vi "Scripting_GetVIClassDependency.vi"(0 "ViRef":refnum<vi>, 5 "error in (no error)":errorcluster) -> (15 "DepVIs":T1[](array[typedef]), 19 "error out":errorcluster)   [LabVIEW 2016]
uses:
  <resource>/Framework/Providers/Open_GDS/ClassProviders/Common/ScriptingFunctions/Scripting_VIClassDependency.ctl
  <resource>/Framework/Providers/Open_GDS/ClassProviders/Common/ScriptingFunctions/SubVIs/Scripting_ViDependencyType.ctl
  <vilib>/Utility/traverseref.llb/TRef TravTarget.ctl
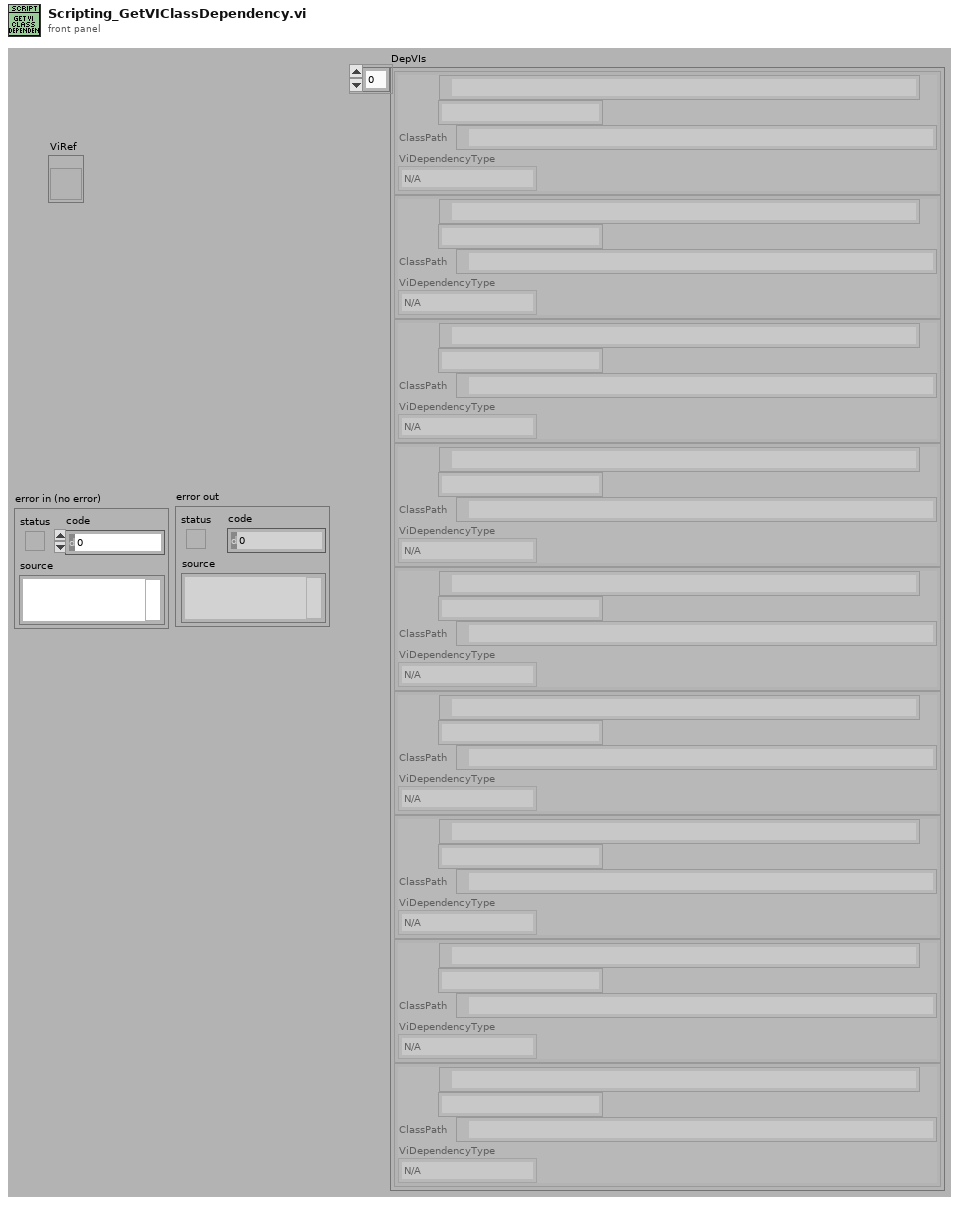
[diagram p1: front panel]
types:
  T1 = typedef "Scripting_VIClassDependency.ctl" = cluster{"VIPath":path, "Class":string, "ClassPath":path, "ViDependencyType":T2}
  T2 = typedef "Scripting_ViDependencyType.ctl" = enum16{"N/A", "Launches"}
  T3 = enum32{"invalid VI type", "Standard VI", "Control VI", "Global VI", "Polymorphic VI", "Configuration VI", "SubSystem", "Facade VI", "Method VI", "Statechart Diagram VI"}
  T4 = enum32{"invalid lock state", "Not Locked", "Locked (No Password)", "Password-protected"}
  T5 = cluster{"ClassControls":refnum<vi>[], "NewClassControl":path, "Diagrams":refnum<vi>[], "DepVIs":T1[]}
  T6 = typedef "TRef TravTarget.ctl" = enum16{"FP", "BD", "Other"}
  T7 = enum32{"not a typedef", "typedef", "strict typedef", "class private data"}
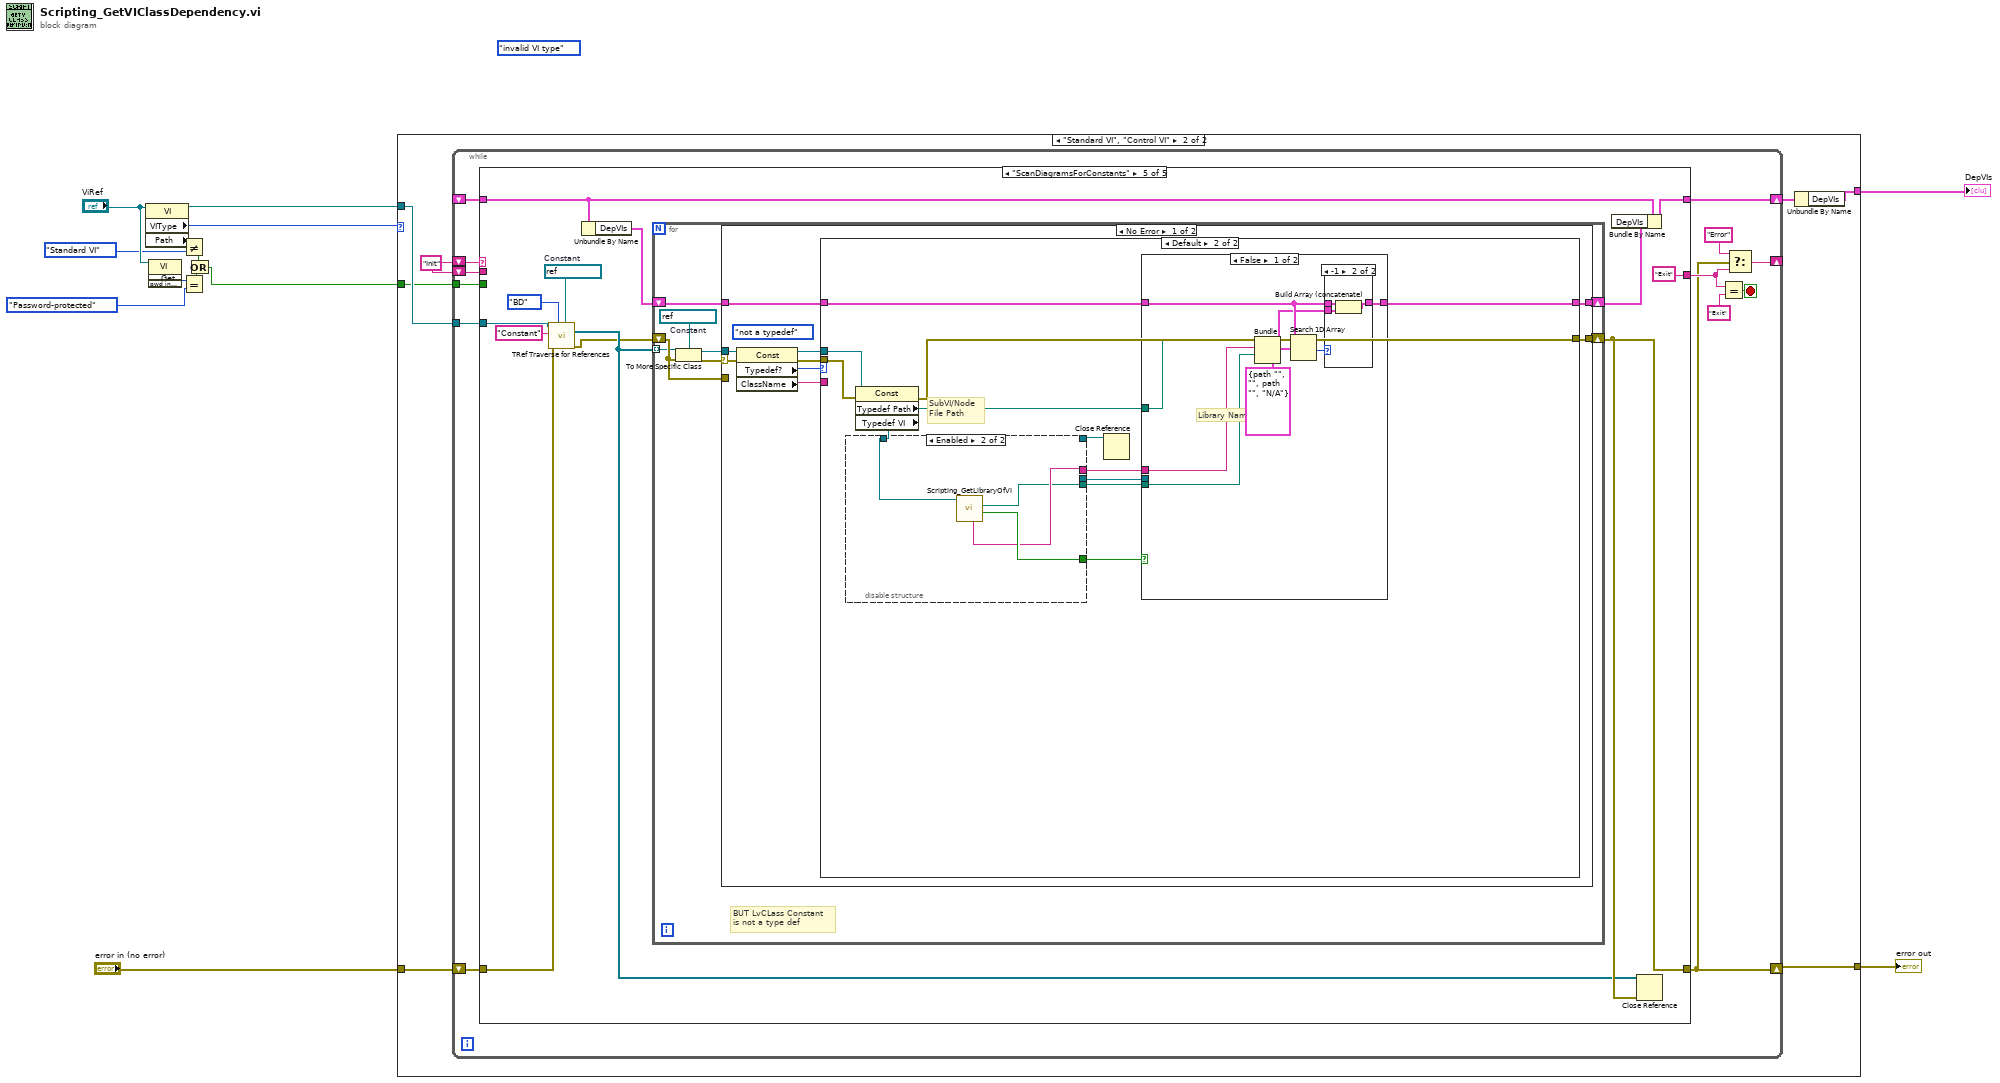
[diagram p0: block diagram]
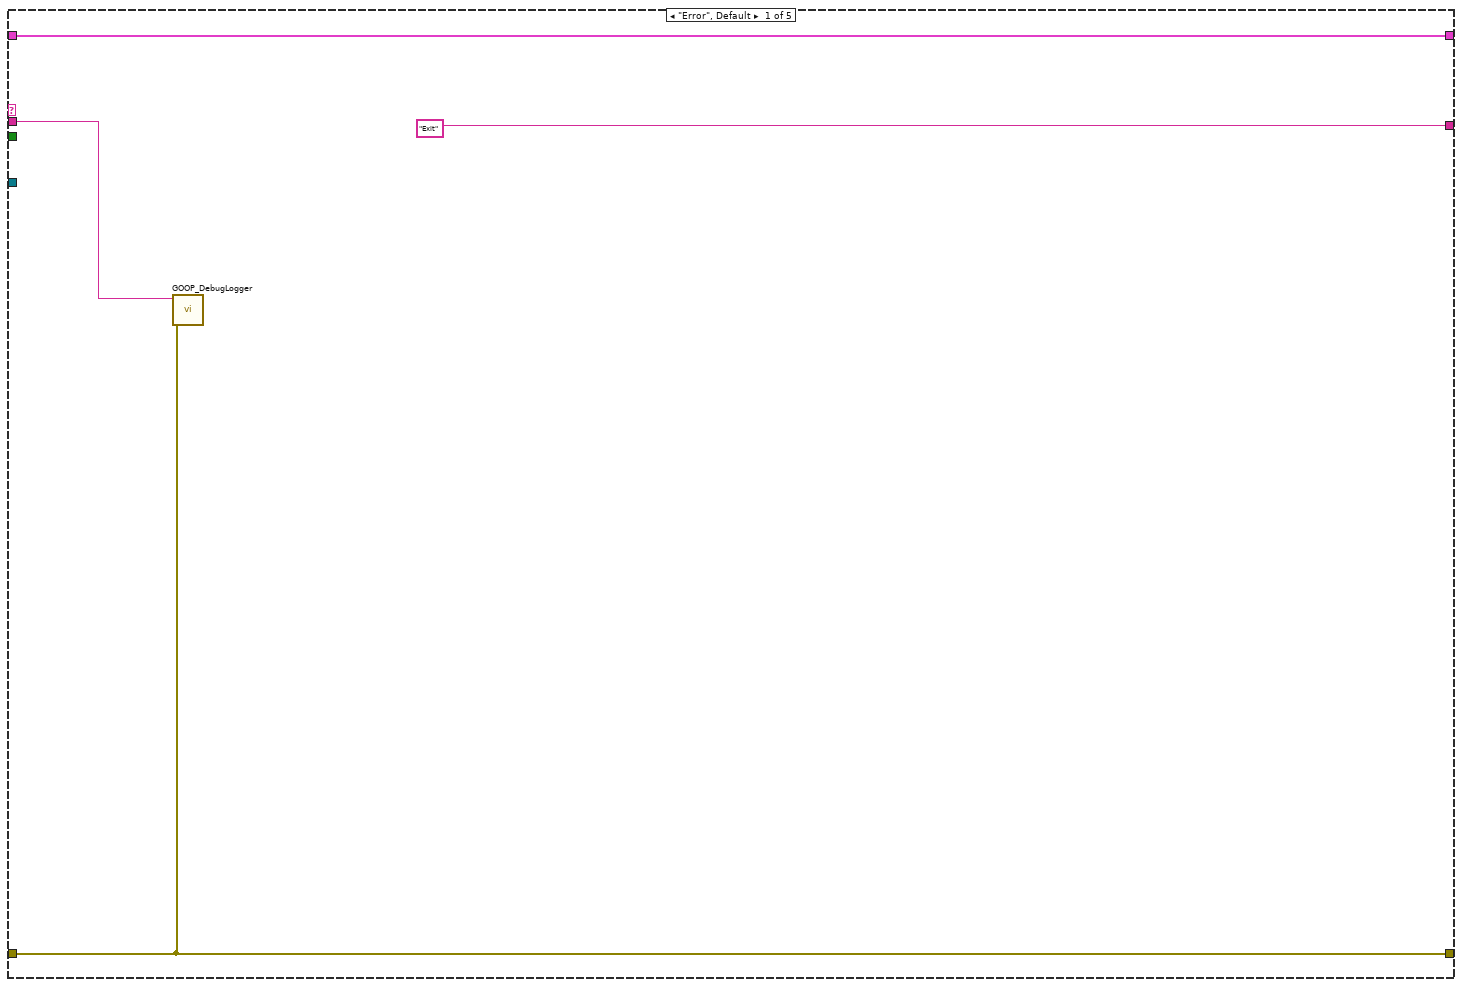
[diagram p3: hidden frame]
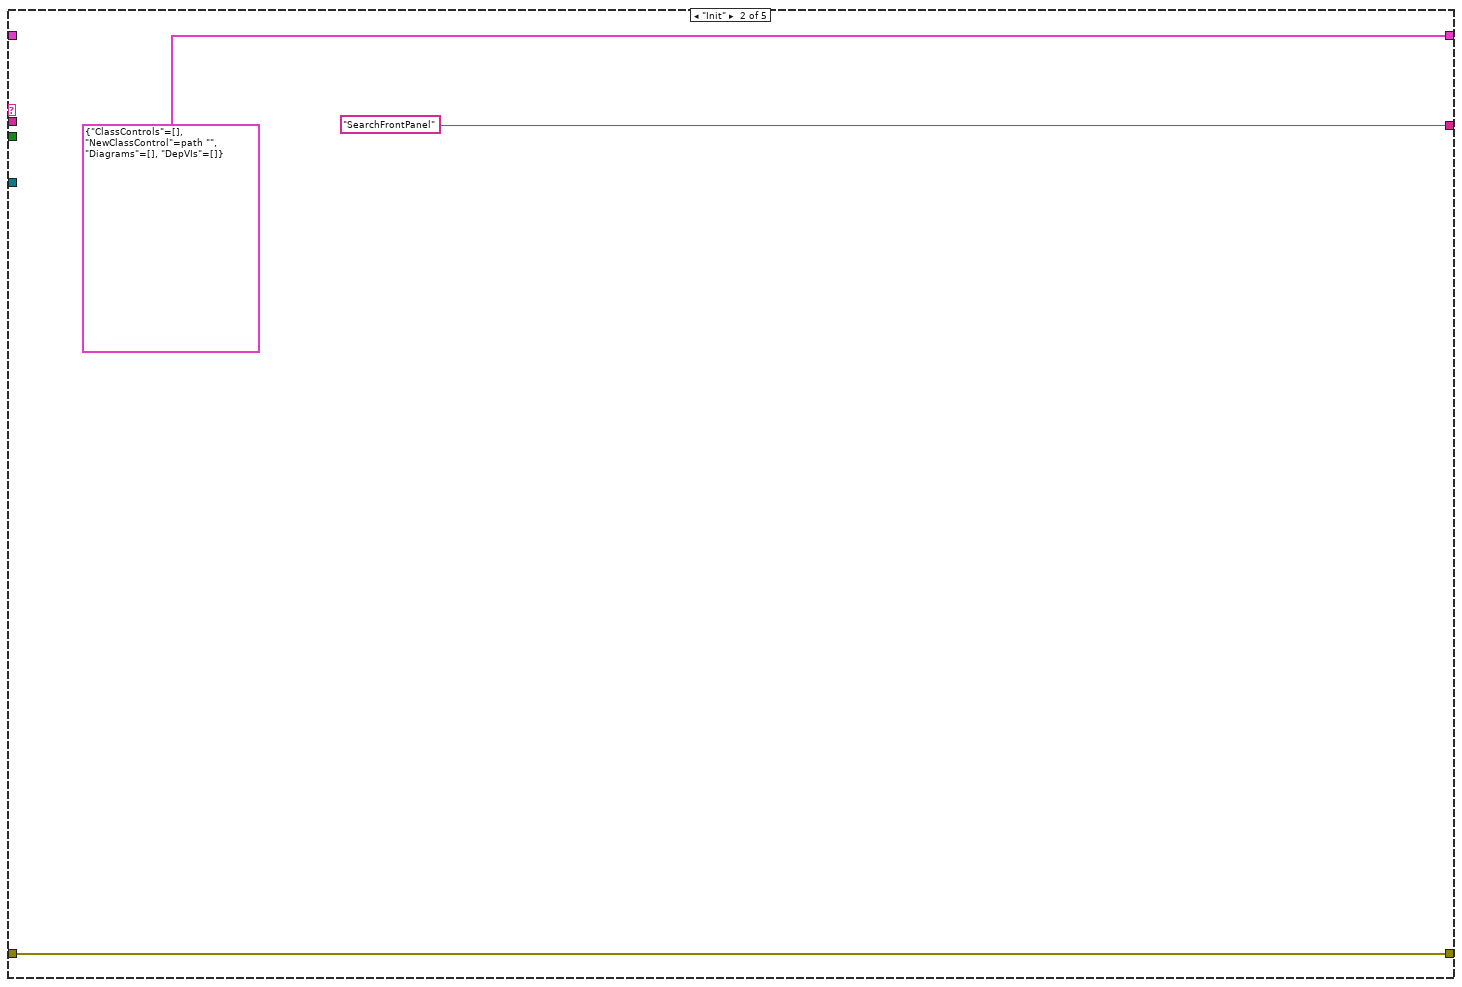
[diagram p4: hidden frame]
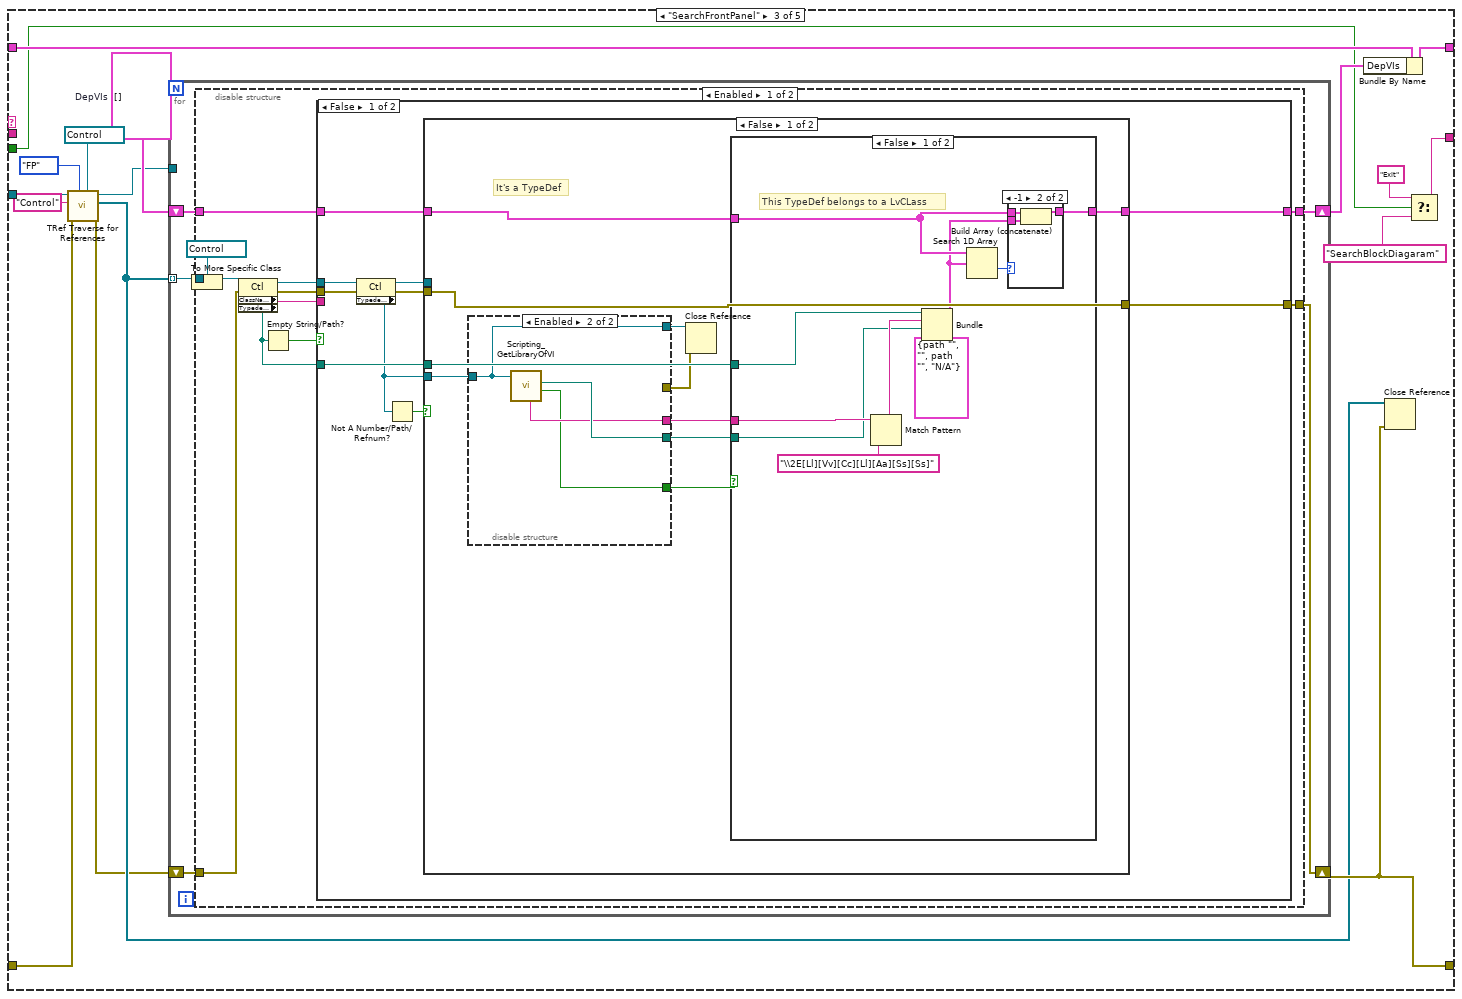
[diagram p5: hidden frame]
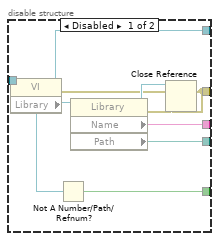
[diagram p6: hidden frame]
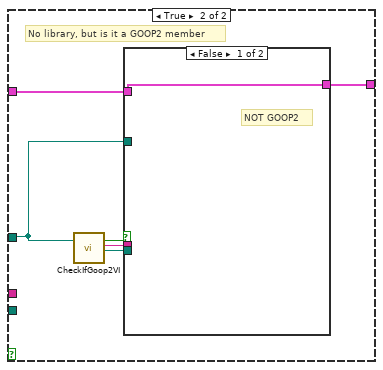
[diagram p8: hidden frame]
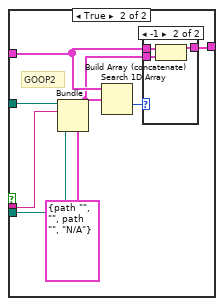
[diagram p9: hidden frame]
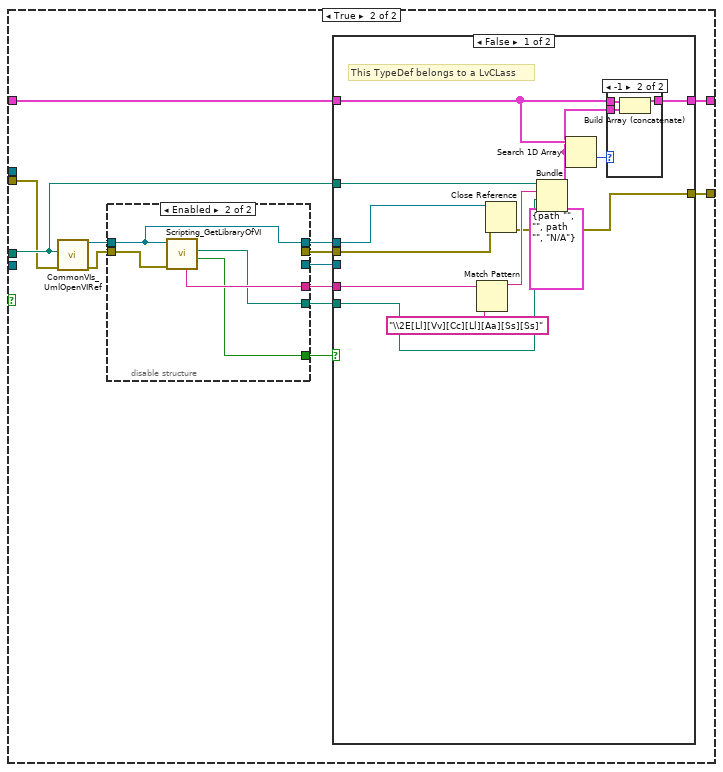
[diagram p11: hidden frame]
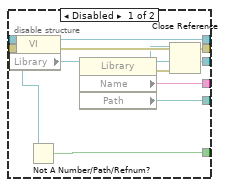
[diagram p12: hidden frame]
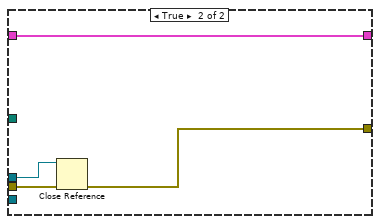
[diagram p14: hidden frame]
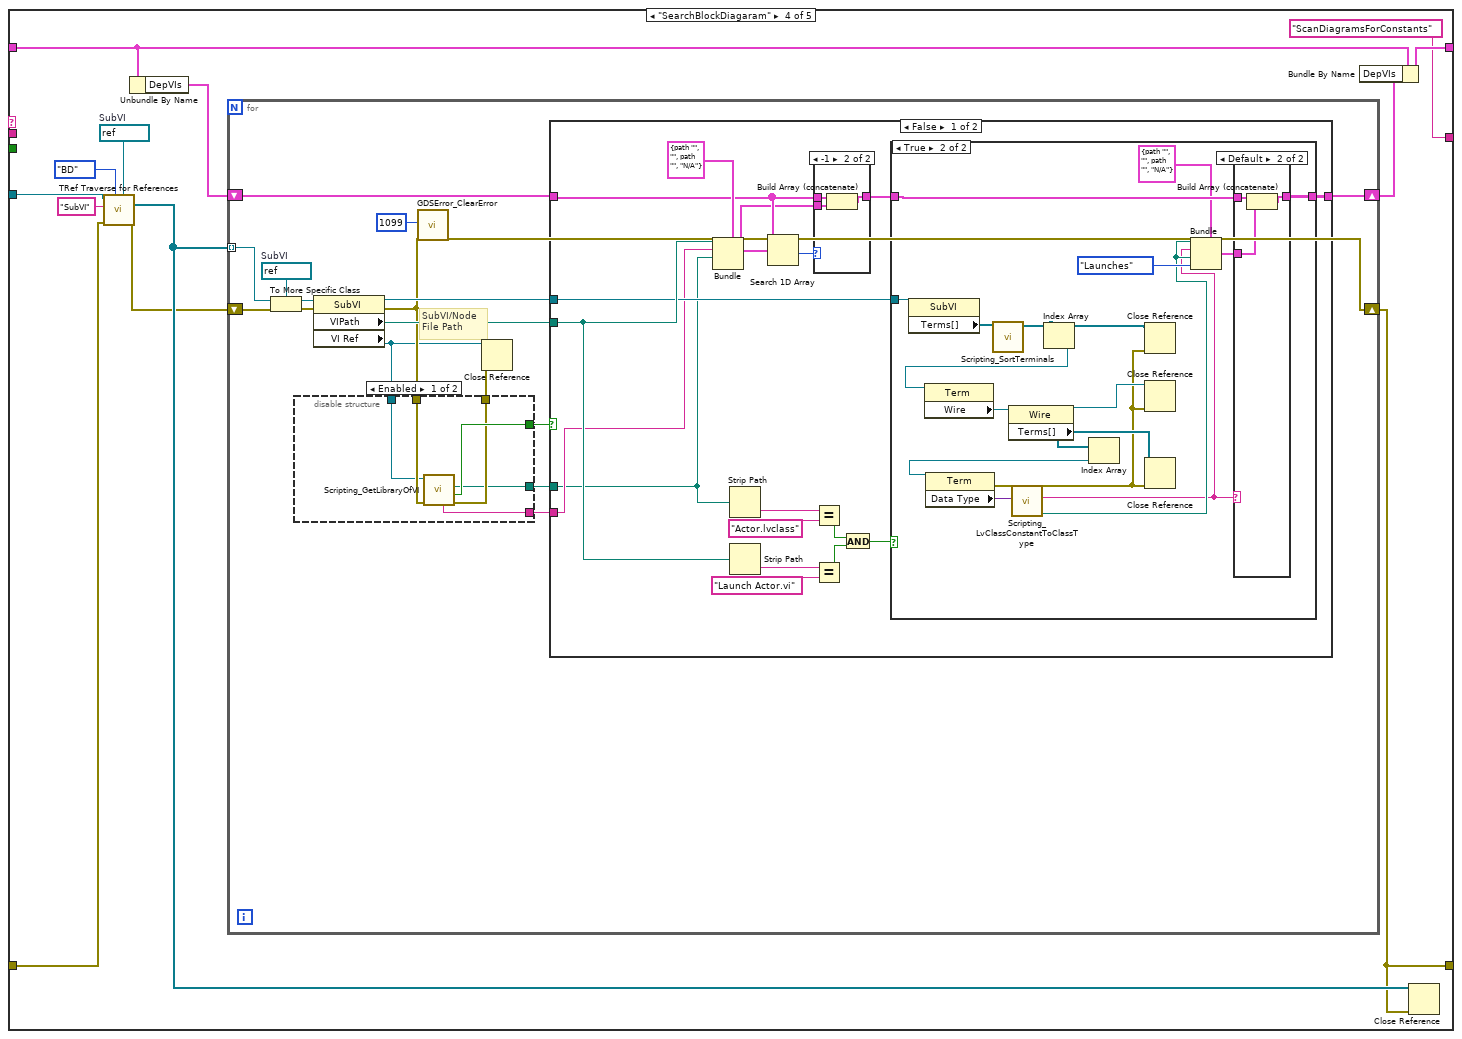
[diagram p17: hidden frame]
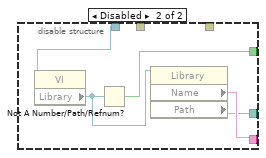
[diagram p18: hidden frame]
diagram:
  (unwired) T3."invalid VI type" ("VI Type")
  n1 = property class="VI" props=["VIType", "Path"](reference="ViRef") -> (reference out=w6:refnum<vi>, "VIType"=w4:T3)  [unwired: 1 in, 2 out]
  n2 = invoke class="VI" method="Lock State.Get"(reference="ViRef") -> ("Get Lock State"=w5:T4)  [unwired: 3 in, 3 out]
  n3 = Not Equal?(x=w4, y=T3."Standard VI") -> (x != y?=w3:bool)
  n4 = Equal?(x=w5, y=T4."Password-protected" ("Lock State")) -> (x = y?=w2:bool)
  n5 = Or(x=w3, y=w2) -> (x .or. y?=w1:bool)
  n6 = case shown="\"Standard VI\", \"Control VI\"" w4 {
    tunnel: "error in (no error)" -> [w13 w20]
    tunnel: w6 -> [_ w19]
    tunnel: [w13 w18] -> w12
    tunnel: w1 -> [_ w17]
    tunnel: [_ w15] -> w9
    frame "invalid VI type", Default {
    }
    frame "Standard VI", "Control VI" {
      w14 = "Init"
      n7 = while {
        shift-right: [w26] -> w18
        shift-left: w20 -> [w33]
        shift-right: [w31] -> _
        shift-left: w14 -> [w32]
        shift-right: [w25] -> w16
        shift-left: _ -> [w24]
        tunnel: w19 -> [w23]
        tunnel: w17 -> [w22]
        shift-left: w14 -> [w21]
        stop <- w30 stop-if-true
        n8 = case shown="\"ScanDiagramsForConstants\"" w32 {
          tunnel: w33 -> [w35 w40 w54 w192 w303]
          tunnel: [w35 w40 w45 w194 w297] -> w26
          tunnel: ["Exit" "SearchFrontPanel" w48 "ScanDiagramsForConstants" "Exit"] -> w27
          tunnel: [w36 T5 {"ClassControls"=[], "NewClassControl"=path "", "Diagrams"=[], "DepVIs"=[]} w50 w204 w307] -> w25
          tunnel: w24 -> [w36 _ w51 w197 w299]
          tunnel: w23 -> [_ _ w53 w200 w304]
          tunnel: w22 -> [_ _ w47 _ _]
          tunnel: w21 -> [w34 _ _ _ _]
          frame "Error", Default {
            n9 = call <resource>:"GOOP_DebugLogger.vi"("error in (no error)"=w35, "State"=w34) -> ()  [unwired: 7 in, 3 out]
          }
          frame "Init" {
          }
          frame "SearchFrontPanel" {
            w52 = T1[] []  # DepVIs
            n10 = call <vilib>:"TRef Traverse for References.vi"("Other Refnum"=refnum<vi> refnum, "Traverse Target"=TRef_TravTarget."FP", "error in (no error)"=w54, "Class Name"="Control", "VI Refnum"=w53) -> ("error out"=w41:errorcluster, "References"=w42:refnum<vi>[], "dup VI Refnum"=w46:refnum<vi>)  [unwired: 3 in, 1 out]
            n11 = for {
              shift-right: [w61] -> w45
              shift-left: w41 -> [w62]
              shift-right: [w60] -> w49
              shift-left: w52 -> [w59]
              tunnel: w42 -> [w58] mode=indexing
              tunnel: w46 -> [_]
              n12 = disable-structure shown="Enabled" {
                disable-tunnel: w62 -> [w72 _]
                disable-tunnel: [w71 _] -> w61
                disable-tunnel: [w68 _] -> w60
                disable-tunnel: w59 -> [w67 _]
                disable-tunnel: w58 -> [w64 _]
                frame Enabled {
                  n13 = To More Specific Class(target class=refnum<vi> refnum ("reference"), reference=w64) -> (specific class reference=w63:refnum<vi>)  [unwired: 1 in, 1 out]
                  n14 = property class="Ctl"(reference=w63, error in=w72) -> (reference out=w66:refnum<vi>, error out=w73:errorcluster, "ClassName"=w74:string, "Typedef Path"=w70:path)
                  n15 = Empty String/Path?(string/path=w70) -> (empty?=w69:bool)
                  n16 = case shown="False" w69 {
                    tunnel: w74 -> [_ _]
                    tunnel: w66 -> [w78 _]
                    tunnel: w73 -> [w76 w190]
                    tunnel: [w84 w190] -> w71
                    tunnel: w70 -> [w83 _]
                    tunnel: [w82 w191] -> w68
                    tunnel: w67 -> [w81 w191]
                    frame False {
                      n17 = property class="Ctl"(reference=w78, error in=w76) -> (reference out=w79:refnum<vi>, error out=w75:errorcluster, "Typedef VI"=w77:refnum<vi>)
                      n18 = Not A Number/Path/Refnum?(number/path/refnum=w77) -> (NaN/Path/Refnum?=w80:bool)
                      n19 = case shown="False" w80 {
                        tunnel: [w88 w149] -> w84
                        tunnel: w79 -> [_ _]
                        tunnel: w83 -> [w94 w147]
                        tunnel: [w93 w150] -> w82
                        tunnel: w81 -> [w92 w151]
                        tunnel: w75 -> [w88 w145]
                        tunnel: w77 -> [w89 _]
                        frame False {
                          # "It's a TypeDef"
                          n20 = disable-structure shown="Enabled" {
                            disable-tunnel: [w103 w104] -> w91
                            disable-tunnel: [w102 w107] -> w90
                            disable-tunnel: w89 -> [w101 w107]
                            disable-tunnel: [w99 w105] -> w87
                            disable-tunnel: [w98 w106] -> w86
                            disable-tunnel: [w95 _] -> w85
                            frame Disabled {
                              n21 = property class="VI"(reference=w101) -> (reference out=w102:refnum<vi>, error out=w95:errorcluster, "Library"=w100:refnum<vi>)  [unwired: 1 in]
                              n22 = Not A Number/Path/Refnum?(number/path/refnum=w100) -> (NaN/Path/Refnum?=w103:bool)
                              n23 = property class="Library"(reference=w100, error in=w95) -> (reference out=w96:refnum<vi>, error out=w97:errorcluster, "Name"=w99:string, "Path"=w98:path)
                              n24 = Close Reference(reference=w96, error in (no error)=w97) -> ()  [unwired: 1 out]
                            }
                            frame Enabled {
                              n25 = call <resource>:"Scripting_GetLibraryOfVI.vi"("VI in"=w107) -> ("NotBelongingToLibrary"=w104:bool, "Path"=w106:path, "Name"=w105:string)  [unwired: 6 in, 2 out]
                            }
                          }
                          n26 = Close Reference(reference=w90, error in (no error)=w85) -> ()  [unwired: 1 out]
                          n27 = case shown="False" w91 {
                            tunnel: w94 -> [w116 w125]
                            tunnel: [w112 w126] -> w93
                            tunnel: w92 -> [w111 w127]
                            tunnel: w87 -> [w109 _]
                            tunnel: w86 -> [w108 _]
                            frame False {
                              # "This TypeDef belongs to a LvCLass"
                              n28 = Match Pattern(string=w109, regular expression="\\2E[Ll][Vv][Cc][Ll][Aa][Ss][Ss]") -> (before substring=w115:string)  [unwired: 1 in, 3 out]
                              n29 = Bundle(cluster=T1 {"VIPath"=path "", "Class"="", "ClassPath"=path "", "ViDependencyType"=enum."N/A"}, "VIPath"=w116, "Class"=w115, "ClassPath"=w108) -> (w110:T1)  [unwired: 1 in]
                              n30 = Search 1D Array(1D array=w111, element=w110) -> (index of element=w113:i32)  [unwired: 1 in]
                              n31 = case shown="-1" w113 {
                                tunnel: [w118 w121] -> w112
                                tunnel: w111 -> [w118 w120]
                                tunnel: w110 -> [_ w119]
                                frame 0, Default {
                                }
                                frame -1 {
                                n32 = Build Array (concatenate)(w120, w119) -> (w121:T1[])
                                }
                              }
                            }
                            frame True {
                              # "No library, but is it a GOOP2 member"
                              n33 = call <resource>:"CheckIfGoop2VI.vi"("ViPath"=w125) -> ("GOOP2Class"=w124:bool, "ClassName"=w123:string, "ClassPath"=w122:path)  [unwired: 15 in, 1 out]
                              n34 = case shown="False" w124 {
                                tunnel: w127 -> [w128 w131]
                                tunnel: [w128 w132] -> w126
                                tunnel: w125 -> [_ w136]
                                tunnel: w123 -> [_ w135]
                                tunnel: w122 -> [_ w129]
                                frame False {
                                # "NOT GOOP2"
                                }
                                frame True {
                                # "GOOP2"
                                n35 = Bundle(cluster=T1 {"VIPath"=path "", "Class"="", "ClassPath"=path "", "ViDependencyType"=enum."N/A"}, "VIPath"=w136, "Class"=w135, "ClassPath"=w129) -> (w130:T1)  [unwired: 1 in]
                                n36 = Search 1D Array(1D array=w131, element=w130) -> (index of element=w133:i32)  [unwired: 1 in]
                                n37 = case shown="-1" w133 {
                                tunnel: [w137 w140] -> w132
                                tunnel: w131 -> [w137 w139]
                                tunnel: w130 -> [_ w138]
                                frame 0, Default {
                                }
                                frame -1 {
                                n38 = Build Array (concatenate)(w139, w138) -> (w140:T1[])
                                }
                                }
                                }
                              }
                            }
                          }
                        }
                        frame True {
                          n39 = call <resource>:"CommonVIs_UmlOpenVIRef.vi"("error in"=w145, "ViPath/ViName"=w147) -> ("error out"=w153:errorcluster, "vi reference"=w144:refnum<vi>)  [unwired: 6 in, 2 out]
                          n40 = disable-structure shown="Enabled" {
                            disable-tunnel: w153 -> [w163 w168]
                            disable-tunnel: [w162 w164] -> w152
                            disable-tunnel: [w161 _] -> w148
                            disable-tunnel: [w160 w165] -> w146
                            disable-tunnel: w144 -> [w159 w165]
                            disable-tunnel: [w156 _] -> w143
                            disable-tunnel: [w155 w167] -> w142
                            disable-tunnel: [w154 w166] -> w141
                            frame Disabled {
                              n41 = property class="VI"(reference=w159, error in=w163) -> (reference out=w160:refnum<vi>, error out=w161:errorcluster, "Library"=w156:refnum<vi>)
                              n42 = Not A Number/Path/Refnum?(number/path/refnum=w156) -> (NaN/Path/Refnum?=w162:bool)
                              n43 = property class="Library"(reference=w156) -> (reference out=w158:refnum<vi>, error out=w157:errorcluster, "Name"=w155:string, "Path"=w154:path)  [unwired: 1 in]
                              n44 = Close Reference(reference=w158, error in (no error)=w157) -> ()  [unwired: 1 out]
                            }
                            frame Enabled {
                              n45 = call <resource>:"Scripting_GetLibraryOfVI.vi"("error in (no error)"=w168, "VI in"=w165) -> ("NotBelongingToLibrary"=w164:bool, "Path"=w166:path, "Name"=w167:string)  [unwired: 5 in, 2 out]
                            }
                          }
                          n46 = case shown="False" w152 {
                            tunnel: w151 -> [w174 w189]
                            tunnel: [w175 w189] -> w150
                            tunnel: [w178 w187] -> w149
                            tunnel: w148 -> [w169 w188]
                            tunnel: w143 -> [_ _]
                            tunnel: w147 -> [w172 _]
                            tunnel: w146 -> [w177 w186]
                            tunnel: w142 -> [w171 _]
                            tunnel: w141 -> [w170 _]
                            frame False {
                              # "This TypeDef belongs to a LvCLass"
                              n47 = Match Pattern(string=w171, regular expression="\\2E[Ll][Vv][Cc][Ll][Aa][Ss][Ss]") -> (before substring=w180:string)  [unwired: 1 in, 3 out]
                              n48 = Close Reference(reference=w177, error in (no error)=w169) -> (error out=w178:errorcluster)
                              n49 = Bundle(cluster=T1 {"VIPath"=path "", "Class"="", "ClassPath"=path "", "ViDependencyType"=enum."N/A"}, "VIPath"=w172, "Class"=w180, "ClassPath"=w170) -> (w173:T1)  [unwired: 1 in]
                              n50 = Search 1D Array(1D array=w174, element=w173) -> (index of element=w176:i32)  [unwired: 1 in]
                              n51 = case shown="-1" w176 {
                                tunnel: [w182 w185] -> w175
                                tunnel: w174 -> [w182 w184]
                                tunnel: w173 -> [_ w183]
                                frame 0, Default {
                                }
                                frame -1 {
                                n52 = Build Array (concatenate)(w184, w183) -> (w185:T1[])
                                }
                              }
                            }
                            frame True {
                              n53 = Close Reference(reference=w186, error in (no error)=w188) -> (error out=w187:errorcluster)
                            }
                          }
                        }
                      }
                    }
                    frame True {
                    }
                  }
                }
                frame Disabled {
                }
              }
            }
            n54 = Bundle By Name(cluster=w51, "DepVIs"=w49) -> (w50:T5)
            n55 = Close Reference(reference=w42, error in (no error)=w45) -> ()  [unwired: 1 out]
            n56 = Select(t="Exit", s=w47, f="SearchBlockDiagaram") -> (s? t:f=w48:string)
          }
          frame "SearchBlockDiagaram" {
            w199 = refnum<vi> refnum  # SubVI
            n57 = call <vilib>:"TRef Traverse for References.vi"("Other Refnum"=w199, "Traverse Target"=TRef_TravTarget."BD", "error in (no error)"=w192, "Class Name"="SubVI", "VI Refnum"=w200) -> ("error out"=w193:errorcluster, "References"=w195:refnum<vi>[])  [unwired: 3 in, 2 out]
            n58 = Unbundle By Name(w197) -> ("DepVIs"=w196:T1[])
            n59 = for {
              shift-right: [w211] -> w194
              shift-left: w193 -> [w212]
              shift-right: [w221] -> w198
              shift-left: w196 -> [w220]
              tunnel: w195 -> [w213] mode=indexing
              w219 = refnum<vi> refnum  # SubVI
              # "SubVI/Node\nFile Path"
              n60 = To More Specific Class(target class=w219, reference=w213, error in=w212) -> (specific class reference=w218:refnum<vi>, error out=w217:errorcluster)
              n61 = property class="SubVI"(reference=w218, error in=w217) -> (reference out=w210:refnum<vi>, error out=w209:errorcluster, "VIPath"=w216:path, "VI Ref"=w206:refnum<vi>)
              n62 = disable-structure shown="Enabled" {
                disable-tunnel: [w227 w230] -> w215
                disable-tunnel: w209 -> [w226 _]
                disable-tunnel: [w225 _] -> w205
                disable-tunnel: [w224 w229] -> w208
                disable-tunnel: [w223 w228] -> w207
                disable-tunnel: w206 -> [w222 w231]
                frame Enabled {
                  n63 = call <resource>:"Scripting_GetLibraryOfVI.vi"("error in (no error)"=w226, "VI in"=w222) -> ("error out"=w225:errorcluster, "NotBelongingToLibrary"=w227:bool, "Path"=w223:path, "Name"=w224:string)  [unwired: 5 in, 1 out]
                }
                frame Disabled {
                  n64 = property class="VI"(reference=w231) -> ("Library"=w232:refnum<vi>)  [unwired: 1 in, 2 out]
                  n65 = Not A Number/Path/Refnum?(number/path/refnum=w232) -> (NaN/Path/Refnum?=w230:bool)
                  n66 = property class="Library"(reference=w232) -> ("Name"=w229:string, "Path"=w228:path)  [unwired: 1 in, 2 out]
                }
              }
              n67 = call <resource>:"GDSError_ClearError.vi"("code"=1099, "error in (no error)"=w209) -> ("error out"=w211:errorcluster)  [unwired: 16 in, 1 out]
              n68 = Close Reference(reference=w206, error in (no error)=w205) -> ()  [unwired: 1 out]
              n69 = case shown="False" w215 {
                tunnel: w216 -> [w241 w278]
                tunnel: w220 -> [w248 w280]
                tunnel: [w235 w279] -> w221
                tunnel: w210 -> [w237 _]
                tunnel: w208 -> [w234 _]
                tunnel: w207 -> [w233 _]
                frame False {
                  n70 = Bundle(cluster=T1 {"VIPath"=path "", "Class"="", "ClassPath"=path "", "ViDependencyType"=enum."N/A"}, "VIPath"=w241, "Class"=w234, "ClassPath"=w233) -> (w247:T1)  [unwired: 1 in]
                  n71 = Strip Path(path=w233) -> (name=w245:string)  [unwired: 1 out]
                  n72 = Strip Path(path=w241) -> (name=w242:string)  [unwired: 1 out]
                  n73 = Search 1D Array(1D array=w248, element=w247) -> (index of element=w246:i32)  [unwired: 1 in]
                  n74 = case shown="-1" w246 {
                    tunnel: [w272 w275] -> w236
                    tunnel: w248 -> [w272 w274]
                    tunnel: w247 -> [_ w273]
                    frame 0, Default {
                    }
                    frame -1 {
                      n75 = Build Array (concatenate)(w274, w273) -> (w275:T1[])
                    }
                  }
                  n76 = Equal?(x=w245, y="Actor.lvclass") -> (x = y?=w240:bool)
                  n77 = Equal?(x=w242, y="Launch Actor.vi") -> (x = y?=w239:bool)
                  n78 = And(x=w240, y=w239) -> (x .and. y?=w238:bool)
                  n79 = case shown="True" w238 {
                    tunnel: w237 -> [_ w267]
                    tunnel: w236 -> [w250 w257]
                    tunnel: [w250 w256] -> w235
                    frame False {
                    }
                    frame True {
                      n80 = property class="SubVI"(reference=w267) -> ("Terms[]"=w266:refnum<vi>[])  [unwired: 1 in, 2 out]
                      n81 = call <resource>:"Scripting_SortTerminals.vi"("Terminals[]"=w266) -> ("TerminalsOut[]"=w258:refnum<vi>[])  [unwired: 8 in, 2 out]
                      n82 = Index Array(array=w258) -> (element=w265:refnum<vi>)  [unwired: 1 in]
                      n83 = property class="Term"(reference=w265) -> ("Wire"=w264:refnum<vi>)  [unwired: 1 in, 2 out]
                      n84 = property class="Wire"(reference=w264) -> (reference out=w260:refnum<vi>, "Terms[]"=w261:refnum<vi>[])  [unwired: 1 in, 1 out]
                      n85 = Index Array(array=w261) -> (element=w263:refnum<vi>)  [unwired: 1 in]
                      n86 = property class="Term"(reference=w263) -> (error out=w259:errorcluster, "Data Type"=w262:variant)  [unwired: 1 in, 1 out]
                      n87 = call <resource>:"Scripting_LvClassConstantToClassType.vi"("Value"=w262) -> ("ClassPath"=w252:path, "JustClassName"=w251:string)  [unwired: 7 in, 2 out]
                      n88 = Close Reference(reference=w258, error in (no error)=w259) -> ()  [unwired: 1 out]
                      n89 = Close Reference(reference=w260, error in (no error)=w259) -> ()  [unwired: 1 out]
                      n90 = Close Reference(reference=w261, error in (no error)=w259) -> ()  [unwired: 1 out]
                      n91 = Bundle(cluster=T1 {"VIPath"=path "", "Class"="", "ClassPath"=path "", "ViDependencyType"=enum."N/A"}, "VIPath"=w252, "Class"=w251, "ClassPath"=w252, "ViDependencyType"=Scripting_ViDependencyType."Launches") -> (w254:T1)
                      n92 = case shown="Default" w251 {
                        tunnel: [w268 w271] -> w256
                        tunnel: w257 -> [w268 w270]
                        tunnel: w254 -> [_ w269]
                        frame "" {
                        }
                        frame Default {
                          n93 = Build Array (concatenate)(w270, w269) -> (w271:T1[])
                        }
                      }
                    }
                  }
                }
                frame True {
                  n94 = call <resource>:"CheckIfGoop2VI.vi"("ViPath"=w278) -> ("GOOP2Class"=w281:bool, "ClassName"=w277:string, "ClassPath"=w276:path)  [unwired: 15 in, 1 out]
                  n95 = case shown="True" w281 {
                    tunnel: w280 -> [w282 w285]
                    tunnel: [w282 w286] -> w279
                    tunnel: w278 -> [_ w290]
                    tunnel: w277 -> [_ w289]
                    tunnel: w276 -> [_ w283]
                    frame False {
                    }
                    frame True {
                      n96 = Bundle(cluster=T1 {"VIPath"=path "", "Class"="", "ClassPath"=path "", "ViDependencyType"=enum."N/A"}, "VIPath"=w290, "Class"=w289, "ClassPath"=w283) -> (w284:T1)  [unwired: 1 in]
                      n97 = Search 1D Array(1D array=w285, element=w284) -> (index of element=w287:i32)  [unwired: 1 in]
                      n98 = case shown="-1" w287 {
                        tunnel: [w291 w294] -> w286
                        tunnel: w285 -> [w291 w293]
                        tunnel: w284 -> [_ w292]
                        frame 0, Default {
                        }
                        frame -1 {
                          n99 = Build Array (concatenate)(w293, w292) -> (w294:T1[])
                        }
                      }
                    }
                  }
                }
              }
            }
            n100 = Bundle By Name(cluster=w197, "DepVIs"=w198) -> (w204:T5)
            n101 = Close Reference(reference=w195, error in (no error)=w194) -> ()  [unwired: 1 out]
          }
          frame "ScanDiagramsForConstants" {
            w302 = refnum<vi> refnum  # Constant
            n102 = call <vilib>:"TRef Traverse for References.vi"("Other Refnum"=w302, "Traverse Target"=TRef_TravTarget."BD", "error in (no error)"=w303, "Class Name"="Constant", "VI Refnum"=w304) -> ("error out"=w295:errorcluster, "References"=w296:refnum<vi>[])  [unwired: 3 in, 2 out]
            n103 = Unbundle By Name(w299) -> ("DepVIs"=w298:T1[])
            n104 = for {
              tunnel: w296 -> [w309] mode=indexing
              shift-right: [w308] -> w297
              shift-left: w295 -> [w311]
              shift-right: [w315] -> w301
              shift-left: w298 -> [w314]
              w313 = refnum<vi> refnum  # Constant
              # "BUT LvCLass Constant \nis not a type def"
              n105 = To More Specific Class(target class=w313, reference=w309, error in=w311) -> (specific class reference=w310:refnum<vi>, error out=w312:errorcluster)
              n106 = case shown="No Error" w312 {
                selector: w312 -> [w321 _]
                tunnel: [w322 w399] -> w308
                tunnel: [w323 w400] -> w315
                tunnel: w314 -> [w324 w400]
                tunnel: w310 -> [w320 _]
                tunnel: w311 -> [_ w399]
                frame No Error {
                  (unwired) T7."not a typedef" ("Is Typedef?")
                  n107 = property class="Const"(reference=w320, error in=w321) -> (reference out=w318:refnum<vi>, error out=w317:errorcluster, "Typedef?"=w319:T7, "ClassName"=w316:string)
                  n108 = case shown="Default" w319 {
                    tunnel: w324 -> [w329 w353]
                    tunnel: [w327 w352] -> w323
                    tunnel: [w326 w351] -> w322
                    tunnel: w318 -> [w325 w350]
                    tunnel: w317 -> [w328 w349]
                    tunnel: w316 -> [w330 _]
                    frame "not a typedef" {
                      n109 = case shown="\"LabVIEWClassConstant\"" w330 {
                        tunnel: w329 -> [w332 w344]
                        tunnel: w328 -> [w331 w337]
                        tunnel: [w332 w343] -> w327
                        tunnel: [w331 w337] -> w326
                        tunnel: w325 -> [_ w342]
                        frame Default {
                        }
                        frame "LabVIEWClassConstant" {
                          w341 = refnum<vi> refnum  # LabVIEWClassConstant
                          n110 = To More Specific Class(target class=w341, reference=w342, error in=w337) -> (specific class reference=w339:refnum<vi>, error out=w340:errorcluster)
                          n111 = property class="LVClassConstant"(reference=w339, error in=w340) -> ("Value"=w338:variant)  [unwired: 2 out]
                          n112 = call <resource>:"Scripting_LvClassConstantToClassType.vi"("Value"=w338) -> ("ClassPath"=w333:path, "JustClassName"=w334:string)  [unwired: 7 in, 2 out]
                          n113 = Bundle By Name(cluster=T1 {"VIPath"=path "", "Class"="", "ClassPath"=path "", "ViDependencyType"=enum."N/A"}, "VIPath"=w333, "Class"=w334, "ClassPath"=w333) -> (w335:T1)
                          n114 = Build Array (concatenate)(w344, w335) -> (w343:T1[])
                        }
                      }
                    }
                    frame Default {
                      # "SubVI/Node\nFile Path"
                      n115 = property class="Const"(reference=w350, error in=w349) -> (error out=w351:errorcluster, "Typedef Path"=w354:path, "Typedef VI"=w356:refnum<vi>)  [unwired: 1 out]
                      n116 = disable-structure shown="Enabled" {
                        disable-tunnel: w356 -> [w363 w367]
                        disable-tunnel: [w362 w366] -> w355
                        disable-tunnel: [w361 _] -> w348
                        disable-tunnel: [w360 _] -> w347
                        disable-tunnel: [w359 w365] -> w346
                        disable-tunnel: [w358 w364] -> w345
                        frame Disabled {
                          n117 = property class="VI"(reference=w363) -> (reference out=w361:refnum<vi>, "Library"=w360:refnum<vi>)  [unwired: 1 in, 1 out]
                          n118 = Not A Number/Path/Refnum?(number/path/refnum=w360) -> (NaN/Path/Refnum?=w362:bool)
                          n119 = property class="Library"(reference=w360) -> (reference out=w357:refnum<vi>, "Name"=w359:string, "Path"=w358:path)  [unwired: 1 in, 1 out]
                          n120 = Close Reference(reference=w357) -> ()  [unwired: 1 in, 1 out]
                        }
                        frame Enabled {
                          n121 = call <resource>:"Scripting_GetLibraryOfVI.vi"("VI in"=w367) -> ("NotBelongingToLibrary"=w366:bool, "Path"=w364:path, "Name"=w365:string)  [unwired: 6 in, 2 out]
                        }
                      }
                      n122 = Close Reference(reference=w348) -> ()  [unwired: 1 in, 1 out]
                      n123 = case shown="False" w355 {
                        tunnel: w347 -> [_ _]
                        tunnel: w354 -> [w374 w382]
                        tunnel: w353 -> [w372 w384]
                        tunnel: [w375 w383] -> w352
                        tunnel: w346 -> [w369 _]
                        tunnel: w345 -> [w368 _]
                        frame False {
                          # "Library Name"
                          n124 = Bundle(cluster=T1 {"VIPath"=path "", "Class"="", "ClassPath"=path "", "ViDependencyType"=enum."N/A"}, "VIPath"=w374, "Class"=w369, "ClassPath"=w368) -> (w371:T1)  [unwired: 1 in]
                          n125 = Search 1D Array(1D array=w372, element=w371) -> (index of element=w370:i32)  [unwired: 1 in]
                          n126 = case shown="-1" w370 {
                            tunnel: [w376 w379] -> w375
                            tunnel: w372 -> [w376 w378]
                            tunnel: w371 -> [_ w377]
                            frame 0, Default {
                            }
                            frame -1 {
                              n127 = Build Array (concatenate)(w378, w377) -> (w379:T1[])
                            }
                          }
                        }
                        frame True {
                          n128 = call <resource>:"CheckIfGoop2VI.vi"("ViPath"=w382) -> ("GOOP2Class"=w385:bool, "ClassName"=w381:string, "ClassPath"=w380:path)  [unwired: 15 in, 1 out]
                          n129 = case shown="True" w385 {
                            tunnel: w384 -> [w386 w389]
                            tunnel: [w386 w390] -> w383
                            tunnel: w382 -> [_ w394]
                            tunnel: w381 -> [_ w393]
                            tunnel: w380 -> [_ w387]
                            frame False {
                            }
                            frame True {
                              n130 = Bundle(cluster=T1 {"VIPath"=path "", "Class"="", "ClassPath"=path "", "ViDependencyType"=enum."N/A"}, "VIPath"=w394, "Class"=w393, "ClassPath"=w387) -> (w388:T1)  [unwired: 1 in]
                              n131 = Search 1D Array(1D array=w389, element=w388) -> (index of element=w391:i32)  [unwired: 1 in]
                              n132 = case shown="0, Default" w391 {
                                tunnel: [w395 w398] -> w390
                                tunnel: w389 -> [w395 w397]
                                tunnel: w388 -> [_ w396]
                                frame 0, Default {
                                }
                                frame -1 {
                                n133 = Build Array (concatenate)(w397, w396) -> (w398:T1[])
                                }
                              }
                            }
                          }
                        }
                      }
                    }
                  }
                }
                frame Error {
                }
              }
            }
            n134 = Bundle By Name(cluster=w299, "DepVIs"=w301) -> (w307:T5)
            n135 = Close Reference(reference=w296, error in (no error)=w297) -> ()  [unwired: 1 out]
          }
        }
        n136 = Equal?(x=w27, y="Exit") -> (x = y?=w30:bool)
        n137 = Select(t="Error", s=w26, f=w27) -> (s? t:f=w31:string)
      }
      n138 = Unbundle By Name(w16) -> ("DepVIs"=w15:T1[])
    }
  }
  "error out" <- w12
  "DepVIs" <- w9
